vi "createNotifier.vi"(8 "error in (no error)":errorcluster, 11 "tcpServerBase in":refnum<class "TcpServerBase.lvclass">) -> (0 "error out":errorcluster, 3 "tcpServerBase out":refnum<class "TcpServerBase.lvclass">)   [LabVIEW 2018, in "TcpServerBase.lvclass"]
doc: "Create notifier reference to send a notification from TCP Server to User everytime TCP Client connects or disconnects."
uses:
  TcpServerBase.lvclass
  TcpServerBase.lvclass/TcpServerBase.ctl
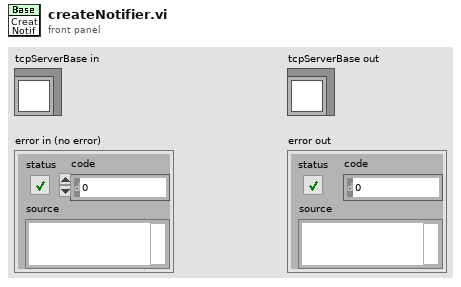
[diagram p1: front panel]
types:
  T1 = cluster{"connectionStatus":bool, "errorSource":string}
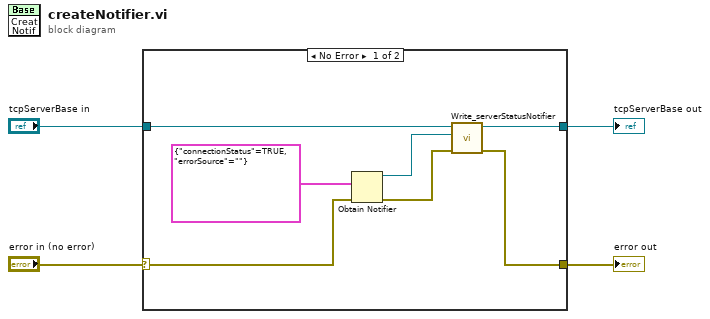
[diagram p0: block diagram]
diagram:
  n1 = case shown="No Error" "error in (no error)" {
    selector: "error in (no error)" -> [w10 w13]
    tunnel: "tcpServerBase in" -> [w9 w12]
    tunnel: [w6 w12] -> w3
    tunnel: [w5 w13] -> w1
    frame No Error {
      n2 = Obtain Notifier(notification data type=T1 {"connectionStatus"=TRUE, "errorSource"=""}, error in (no error)=w10) -> (notifier out=w7:refnum<notifier>, error out=w8:errorcluster)  [unwired: 2 in, 1 out]
      n3 = call "Write_serverStatusNotifier.vi"("error in (no error)"=w8, "serverStatusNotifier"=w7, "TcpServerBase in"=w9) -> ("error out"=w5:errorcluster, "TcpServerBase out"=w6:refnum<class "TcpServerBase.lvclass">)  [unwired: 7 in]
    }
    frame Error {
    }
  }
  "error out" <- w1
  "tcpServerBase out" <- w3
